vi "signal_generation_v1.vi"() -> ()   [LabVIEW 2020]
uses:
  <vilib>/DAQmx/write.llb/DAQmx Write (Analog Wfm 1Chan NSamp).vi
  <vilib>/DAQmx/read.llb/DAQmx Read (Analog Wfm 1Chan NSamp).vi
  <vilib>/DAQmx/create/channels.llb/DAQmx Create Channel (AO-Voltage-Basic).vi
  <vilib>/DAQmx/configure/timing.llb/DAQmx Timing (Sample Clock).vi
  <vilib>/Utility/file.llb/Read Delimited Spreadsheet (DBL).vi
  <vilib>/DAQmx/create/channels.llb/DAQmx Create Channel (AI-Voltage-Basic).vi
  <vilib>/DAQmx/miscellaneous.llb/DAQmx Fill In Error Info.vi
  <resource>/objmgr/daqmx.rc
panel:
  in  "Combo Box":string(combo)
  out "file location for save":path
  out "Ivol":dynamicdata(graph)
  in  "file to run":path=path "C:/Users/Puja/Desktop/Labview(PC)/Input_Signal/Sine_wave_data_without_time/data1_w1_NT_1per.txt"
  out "Input":waveform(dbl)(graph)
  in  "error in":errorcluster
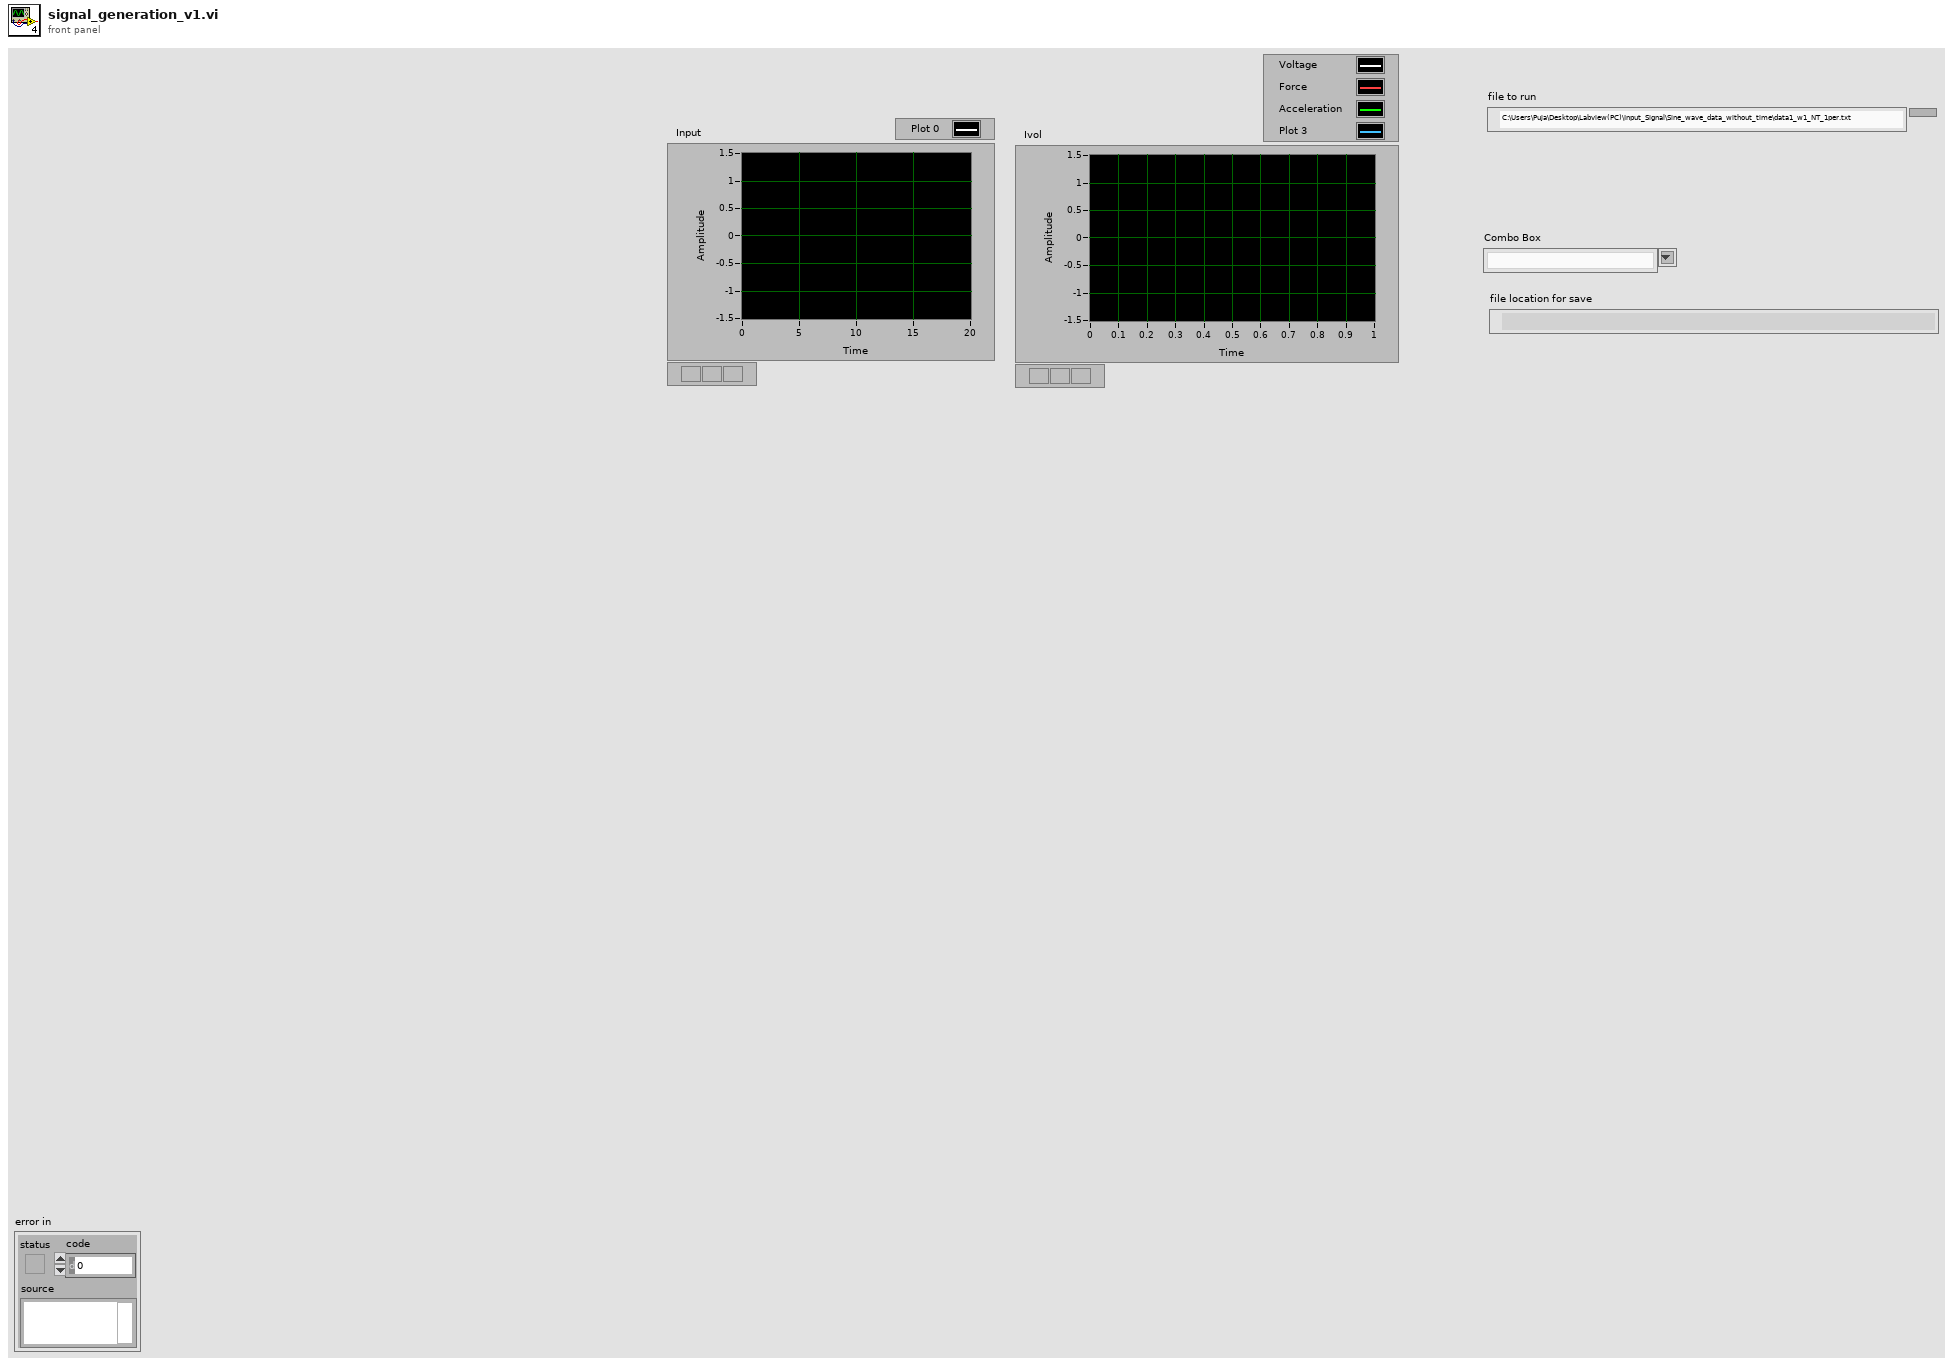
[diagram p1: front panel]
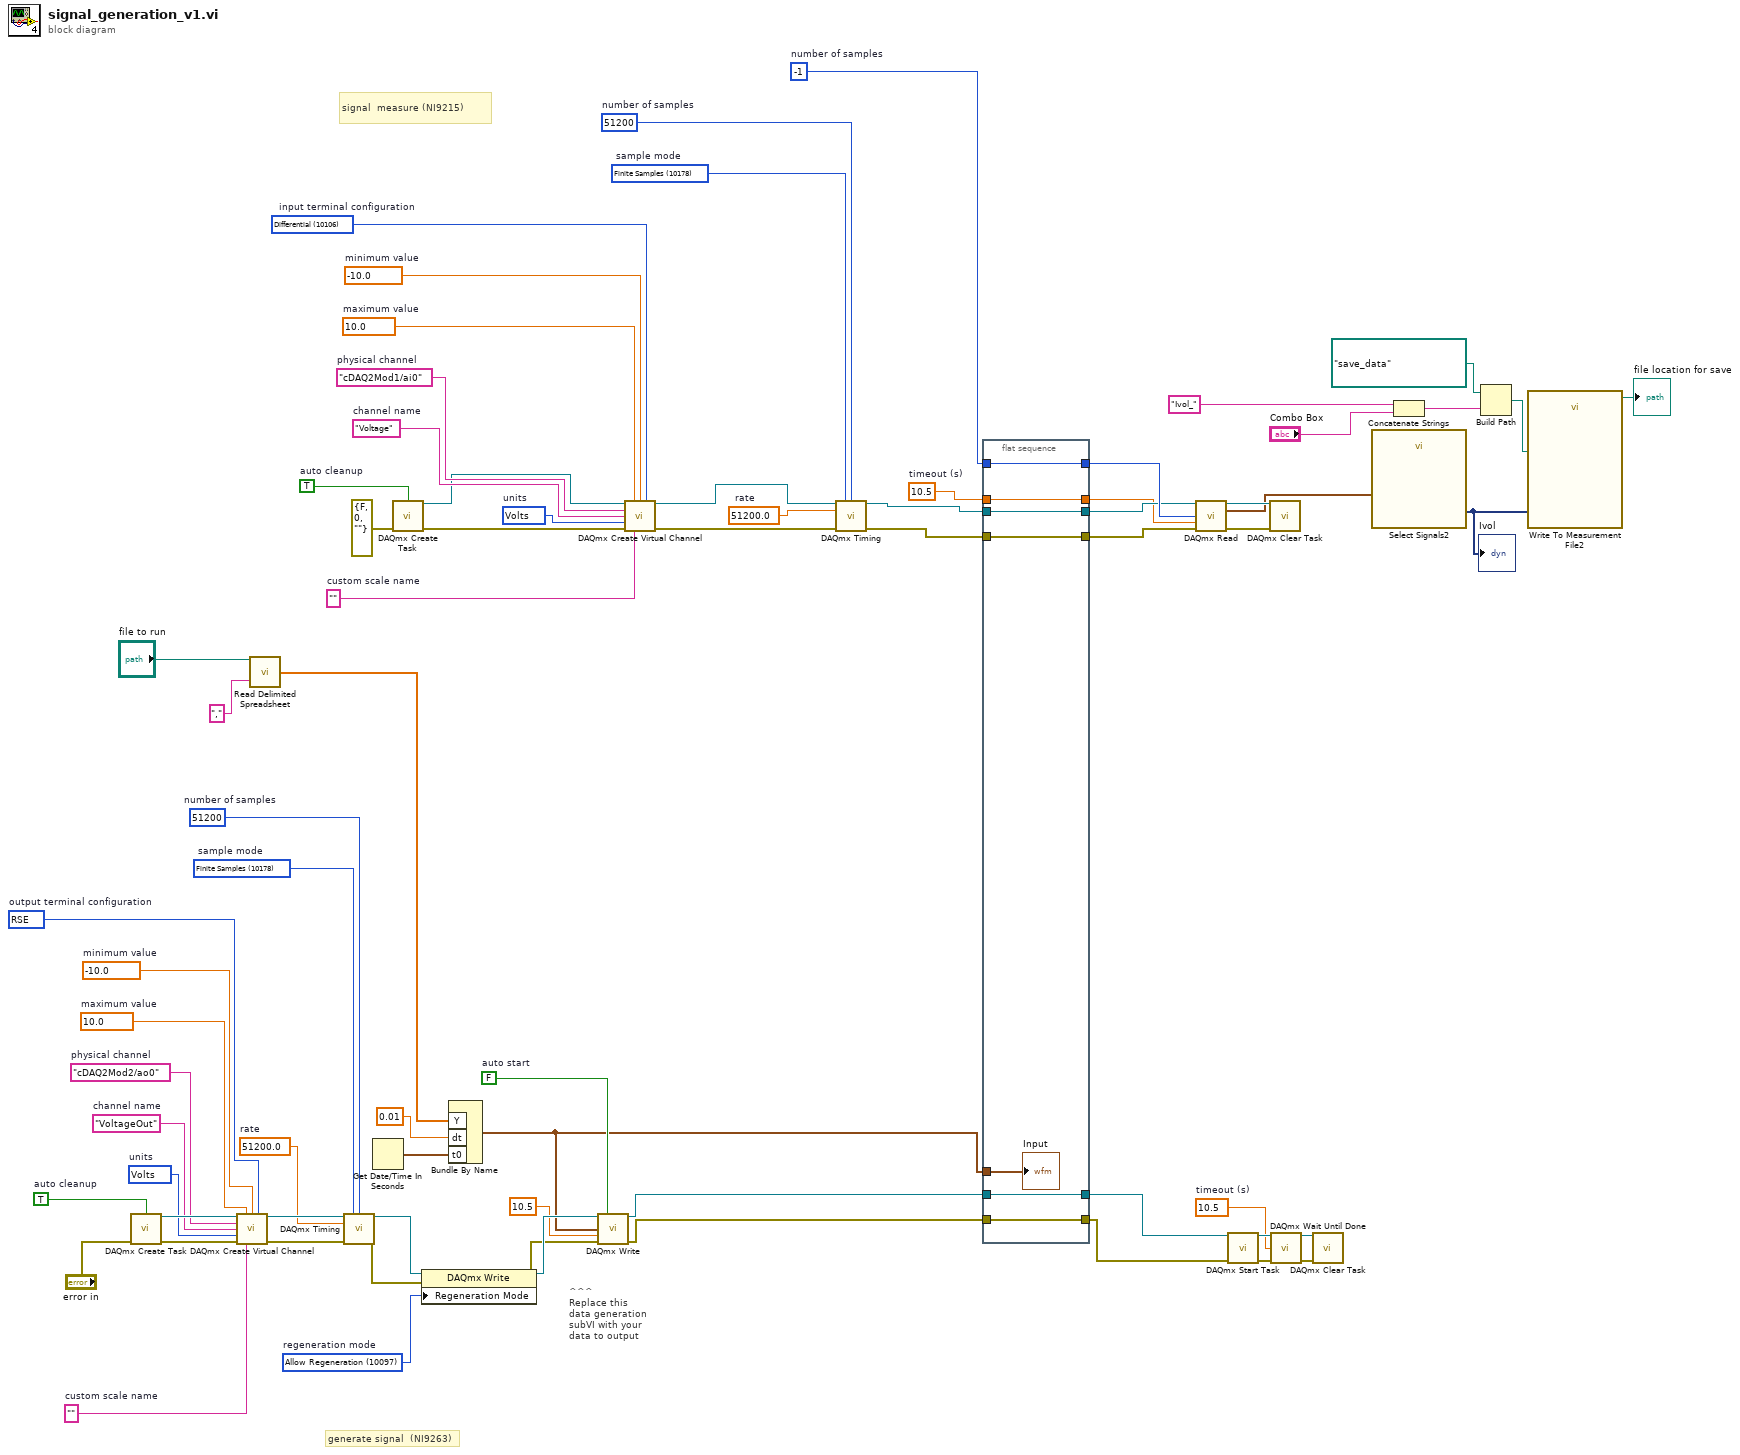
[diagram p0: block diagram]
diagram:
  w12 = 10178 items=["Finite Samples"=10178, "Continuous Samples"=10123, "Hardware Timed Single Point"=12522]  # sample mode
  w11 = 51200  # number of samples
  w10 = 51200.0  # rate
  w22 = 10106 items=["default"=-1, "RSE"=10083, "NRSE"=10078, "Differential"=10106, "Pseudodifferential"=12529]  # input terminal configuration
  w23 = 10348 items=["Volts"=10348, "From Custom Scale"=10065]  # units
  w24 = "Voltage"  # channel name
  w25 = ""  # custom scale name
  w26 = -10.0  # minimum value
  w27 = 10.0  # maximum value
  w28 = "cDAQ2Mod1/ai0"  # physical channel
  w34 = TRUE  # auto cleanup
  w2 = 10.5  # timeout (s)
  w33 = -1  # number of samples
  w48 = 10097 items=["Allow Regeneration"=10097, "Do Not Allow Regeneration"=10158]  # regeneration mode
  w50 = 10178 items=["Finite Samples"=10178, "Continuous Samples"=10123, "Hardware Timed Single Point"=12522]  # sample mode
  w51 = 51200  # number of samples
  w52 = 51200.0  # rate
  w55 = 10083 items=["Default"=-1, "RSE"=10083, "Differential"=10106, "Pseudodifferential"=12529]  # output terminal configuration
  w56 = 10348 items=["Volts"=10348, "From Custom Scale"=10065]  # units
  w57 = "VoltageOut"  # channel name
  w59 = ""  # custom scale name
  w60 = -10.0  # minimum value
  w61 = 10.0  # maximum value
  w62 = "cDAQ2Mod2/ao0"  # physical channel
  w64 = TRUE  # auto cleanup
  w68 = 10.5  # timeout (s)
  w72 = FALSE  # auto start
  # "signal  measure (NI9215)"
  # "generate signal  (NI9263)"
  # "^^^\nReplace this\ndata generation\nsubVI with your\ndata to output"
  n1 = call <vilib>:"DAQmx Create Task.vi"("auto cleanup"=w64, "error in"="error in") -> ("task out"=w63:refnum<k21>, "error out"=w65:errorcluster)  [unwired: 12 in]
  n2 = call-poly <vilib>:"DAQmx Create Virtual Channel.vi"("task in"=w63, "maximum value"=w61, "minimum value"=w60, "output terminal configuration"=w55, "physical channels"=w62, "name to assign"=w57, "units"=w56, "error in"=w65, "custom scale name"=w59) -> ("task out"=w53:refnum<k21>, "error out"=w58:errorcluster)  [unwired: 5 in]
  n3 = call-poly <vilib>:"Read Delimited Spreadsheet.vi"("file path (dialog if empty)"="file to run", "delimiter (\\t)"=",") -> ("first row"=w38:dbl[])  [unwired: 8 in, 5 out]
  n4 = call-poly <vilib>:"DAQmx Timing.vi"("task/channels in"=w53, "sample mode"=w50, "samples per channel"=w51, "rate"=w52, "error in"=w58) -> ("task out"=w49:refnum<k21>, "error out"=w54:errorcluster)  [unwired: 9 in]
  n5 = Get Date/Time In Seconds() -> (seconds since 1Jan1904=w36:timestamp)
  n6 = call <vilib>:"DAQmx Create Task.vi"("auto cleanup"=w34, "error in"=errorcluster {"status"=FALSE, "code"=0, "source"=""}) -> ("task out"=w21:refnum<k21>, "error out"=w20:errorcluster)  [unwired: 12 in]
  n7 = property class="DAQmx Write"(reference=w49, error in=w54, "Regeneration Mode"=w48) -> (reference out=w47:refnum<k21>, error out=w46:errorcluster)
  n8 = Bundle By Name("Y"=w38, "dt"=0.01, "t0"=w36) -> (w32:waveform(dbl))  [unwired: 1 in]
  n9 = call-poly <vilib>:"DAQmx Write.vi"("task/channels in"=w47, "auto start"=w72, "data"=w32, "timeout"=10.5, "error in"=w46) -> ("task out"=w44:refnum<k21>, "error out"=w42:errorcluster)  [unwired: 8 in, 1 out]
  n10 = call-poly <vilib>:"DAQmx Create Virtual Channel.vi"("task in"=w21, "maximum value"=w27, "minimum value"=w26, "input terminal configuration"=w22, "physical channels"=w28, "name to assign"=w24, "units"=w23, "error in"=w20, "custom scale name"=w25) -> ("task out"=w9:refnum<k21>, "error out"=w8:errorcluster)  [unwired: 5 in]
  n11 = call-poly <vilib>:"DAQmx Timing.vi"("task/channels in"=w9, "sample mode"=w12, "samples per channel"=w11, "rate"=w10, "error in"=w8) -> ("task out"=w7:refnum<k21>, "error out"=w5:errorcluster)  [unwired: 9 in]
  n12 = flat-sequence {
    tunnel: w44 -> [w79]
    tunnel: w42 -> [w78]
    tunnel: w33 -> [w77]
    tunnel: w32 -> [w76]
    tunnel: [w79] -> w43
    tunnel: [w78] -> w41
    tunnel: [w77] -> w29
    tunnel: w7 -> [w75]
    tunnel: [w75] -> w6
    tunnel: [w74] -> w4
    tunnel: w5 -> [w74]
    tunnel: [w73] -> w3
    tunnel: w2 -> [w73]
    frame #0 {
      "Input" <- w76
    }
  }
  n13 = call-poly <vilib>:"DAQmx Read.vi"("task/channels in"=w6, "number of samples per channel"=w29, "timeout"=w3, "error in"=w4) -> ("task out"=w31:refnum<k21>, "data"=w19:waveform(dbl), "error out"=w30:errorcluster)  [unwired: 9 in]
  n14 = call <vilib>:"DAQmx Start Task.vi"("task/channels in"=w43, "error in"=w41) -> ("task out"=w71:refnum<k21>, "error out"=w70:errorcluster)  [unwired: 12 in]
  n15 = call <vilib>:"DAQmx Clear Task.vi"("task in"=w31, "error in"=w30) -> ()  [unwired: 13 in, 1 out]
  n16 = call <vilib>:"DAQmx Wait Until Done.vi"("task/channels in"=w71, "timeout (sec)"=w68, "error in"=w70) -> ("task out"=w67:refnum<k21>, "error out"=w69:errorcluster)  [unwired: 11 in]
  n17 = call <vilib>:"DAQmx Clear Task.vi"("task in"=w67, "error in"=w69) -> ()  [unwired: 13 in, 1 out]
  n18 = call "Select Signals2"("Signals"=w19) -> ("Signal Out"=w1:dynamicdata)  [unwired: 9 in, 1 out]
  "Ivol" <- w1
  n19 = Concatenate Strings("Ivol_", "Combo Box") -> (w16:string)
  n20 = Build Path(base path=path "save_data", name or relative path=w16) -> (appended path=w15:path)
  n21 = call "Write To Measurement File2"("Signals"=w1, "Filename"=w15) -> ("Filename Out"=→"file location for save":path)  [unwired: 15 in, 2 out]
